vi "Measure.vi"(8 "error in":errorcluster, 11 "DAQ970 in":refnum<class "DAQ970.lvclass">) -> (0 "error out":errorcluster, 3 "DAQ970 out":refnum<class "DAQ970.lvclass">)   [LabVIEW 2019, in "DAQ970.lvlib" / "DAQ970.lvclass"]
uses:
  Library/DAQ970.lvclass
  C:/Users/Public/Documents/Development/builds/Instruments/Instruments.lvlibp/Library/Instruments.lvclass
  Custom Controls/Measurement Modes.ctl
  builds/Instruments/Instruments.lvlibp/Accessors/Read dt.vi
  builds/Instruments/Instruments.lvlibp/Accessors/Write Measured.vi
  builds/Instruments/Instruments.lvlibp/Library/Instruments.lvclass
panel:
  in  "Measurement Types":T1
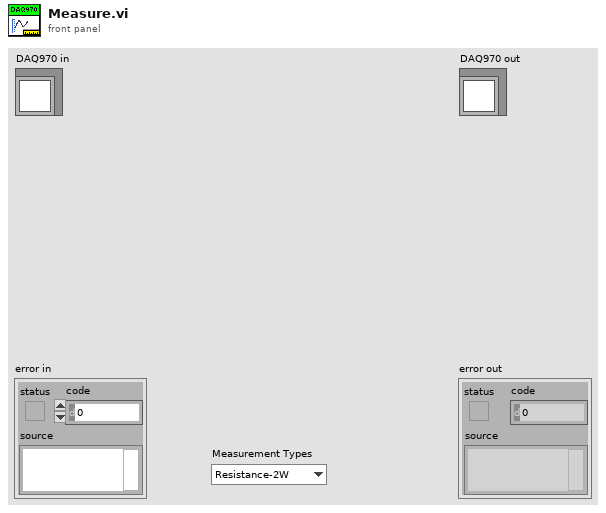
[diagram p1: front panel]
types:
  T1 = typedef "DAQ970.lvlib/DAQ970.lvclass/Measurement Modes.ctl" = enum16{"Resistance-2W", "Resistance-4W", "Capacitance", "Diode", "DC_Current", "DC_Voltage", "Digital_In", "Digital_Out"}
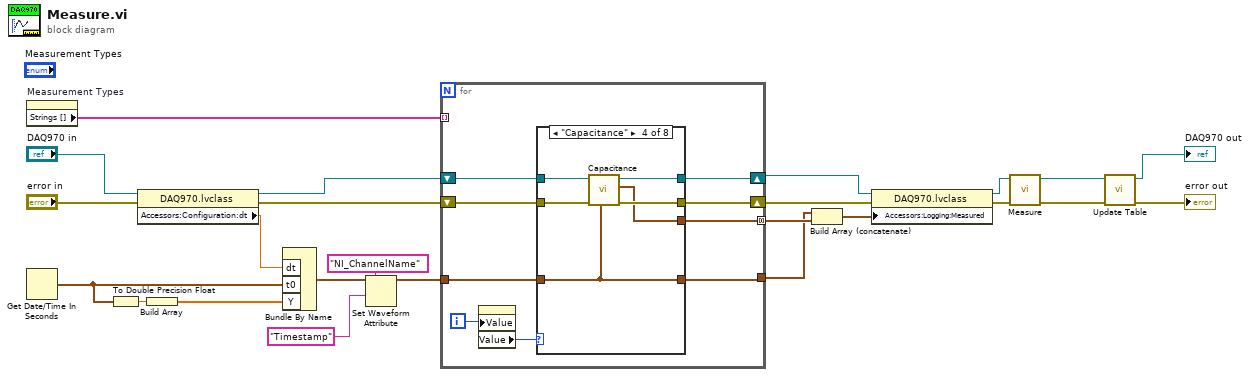
[diagram p0: block diagram]
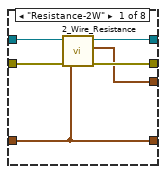
[diagram p2: hidden frame]
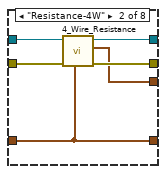
[diagram p3: hidden frame]
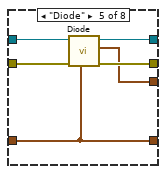
[diagram p5: hidden frame]
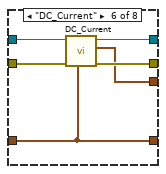
[diagram p6: hidden frame]
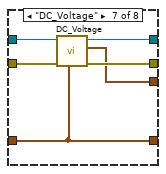
[diagram p7: hidden frame]
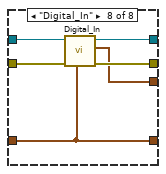
[diagram p8: hidden frame]
diagram:
  n1 = property on="Measurement Types" class="Enum (strict)"() -> ("Strings []"=w5:string[])  [unwired: 2 in, 2 out]
  n2 = Get Date/Time In Seconds() -> (seconds since 1Jan1904=w13:timestamp)
  n3 = To Double Precision Float(number=w13) -> (double precision float=w12:dbl)
  n4 = property class="DAQ970.lvclass"(reference="DAQ970 in", error in="error in") -> (reference out=w21:refnum<class "DAQ970.lvclass">, error out=w20:errorcluster, "Accessors:Configuration:dt"=w22:dbl)
  n5 = Build Array(w12) -> (w14:dbl[])
  n6 = Bundle By Name("dt"=w22, "t0"=w13, "Y"=w14) -> (w15:waveform(dbl))  [unwired: 1 in]
  n7 = Set Waveform Attribute(5:"Timestamp" ("name"), 6:"NI_ChannelName" ("name"), 7:w15) -> (3:w11:waveform(dbl))  [unwired: 1 in, 2 out]
  n8 = for {
    shift-right: [w31] -> w18
    shift-left: w21 -> [w33]
    shift-right: [w30] -> w19
    shift-left: w20 -> [w32]
    tunnel: w11 -> [w29]
    tunnel: [w28] -> w8 mode=concatenating
    tunnel: [w27] -> w7
    tunnel: w5 -> [_] mode=indexing
    i -> [w26]
    n9 = property on="Measurement Types" class="Enum (strict)"("Value"=w26) -> ("Value"=w25:T1)  [unwired: 2 in, 2 out]
    n10 = case shown="\"Capacitance\"" w25 {
      tunnel: w33 -> [w39 w44 w47 w54 w59 w65 w72 w77]
      tunnel: w32 -> [w38 w45 w46 w51 w60 w66 w71 w78]
      tunnel: [w37 w43 w47 w53 w58 w64 w69 w76] -> w31
      tunnel: [w36 w42 w46 w52 w57 w63 w70 w75] -> w30
      tunnel: w29 -> [w35 w40 w48 w50 w56 w62 w68 w73]
      tunnel: [w34 w41 _ w49 w55 w61 w67 w74] -> w28
      tunnel: [w35 w40 w48 w50 w56 w62 w68 w73] -> w27
      frame "Resistance-2W" {
        n11 = call "2_Wire_Resistance.vi"("Waveform_Template"=w35, "error in"=w38, "DAQ970 in"=w39) -> ("error out"=w36:errorcluster, "Resistive_Measurement"=w34:waveform(dbl)[], "DAQ970 out"=w37:refnum<class "DAQ970.lvclass">)  [unwired: 6 in]
      }
      frame "Resistance-4W" {
        n12 = call "4_Wire_Resistance.vi"("Waveform_Template"=w40, "error in"=w45, "DAQ970 in"=w44) -> ("error out"=w42:errorcluster, "Resistive_Measurement"=w41:waveform(dbl)[], "DAQ970 out"=w43:refnum<class "DAQ970.lvclass">)  [unwired: 6 in]
      }
      frame "Digital_Out" {
      }
      frame "Capacitance" {
        n13 = call "Capacitance.vi"("Waveform_Template"=w50, "error in"=w51, "DAQ970 in"=w54) -> ("error out"=w52:errorcluster, "Capacitive_Measurement"=w49:waveform(dbl)[], "DAQ970 out"=w53:refnum<class "DAQ970.lvclass">)  [unwired: 6 in]
      }
      frame "Diode" {
        n14 = call "Diode.vi"("Waveform_Template"=w56, "error in"=w60, "DAQ970 in"=w59) -> ("error out"=w57:errorcluster, "Diode_Measurement"=w55:waveform(dbl)[], "DAQ970 out"=w58:refnum<class "DAQ970.lvclass">)  [unwired: 6 in]
      }
      frame "DC_Current" {
        n15 = call "DC_Current.vi"("Waveform_Template"=w62, "error in"=w66, "DAQ970 in"=w65) -> ("error out"=w63:errorcluster, "DC_Current_Measurement"=w61:waveform(dbl)[], "DAQ970 out"=w64:refnum<class "DAQ970.lvclass">)  [unwired: 6 in]
      }
      frame "DC_Voltage" {
        n16 = call "DC_Voltage.vi"("Waveform_Template"=w68, "error in"=w71, "DAQ970 in"=w72) -> ("error out"=w70:errorcluster, "DC_Voltage_Measurement"=w67:waveform(dbl)[], "DAQ970 out"=w69:refnum<class "DAQ970.lvclass">)  [unwired: 6 in]
      }
      frame "Digital_In" {
        n17 = call "Digital_In.vi"("Waveform_Template"=w73, "error in"=w78, "DAQ970 in"=w77) -> ("error out"=w75:errorcluster, "DC_Voltage_Measurement"=w74:waveform(dbl)[], "DAQ970 out"=w76:refnum<class "DAQ970.lvclass">)  [unwired: 6 in]
      }
    }
  }
  n18 = Build Array (concatenate)(w7, w8) -> (w6:waveform(dbl)[])
  n19 = property class="DAQ970.lvclass"(reference=w18, error in=w19, "Accessors:Logging:Measured"=w6) -> (reference out=w17:refnum<class "DAQ970.lvclass">, error out=w16:errorcluster)
  n20 = call-parent "Measure.vi"("error in"=w16, "Instruments in"=w17) -> ("error out"=w3:errorcluster, "Instruments out"=w4:refnum<class "DAQ970.lvclass">)  [unwired: 8 in]
  n21 = call "Update Table.vi"("error in (no error)"=w3, "DAQ970 in"=w4) -> ("error out"=→"error out":errorcluster, "DAQ970 out"=→"DAQ970 out":refnum<class "DAQ970.lvclass">)  [unwired: 8 in]
